vi "Do.vi"(8 "error in":errorcluster, 10 "Actor in":refnum<class "Actor.lvclass">, 11 "Update Device Configuration MSG":refnum<class "Update Device Configuration MSG.lvclass">) -> (0 "error out":errorcluster, 2 "Actor out":refnum<class "Actor.lvclass">)   [LabVIEW 2014, in "Controller.lvlib" / "Update Device Configuration MSG.lvclass"]
doc: "(<B>Filename</B>: Actor Framework.lvlib:Message.lvclass:Do.vi)\n\nDefines what a message does when it is received by an actor. Generally, a message instructs an actor to invoke one of its methods. By default, this method does nothing. A child class must override it to define behavior. Create a child class by using the Actor Framework Message Maker dialog box."
uses:
  Update Device Configuration MSG.lvclass
  <vilib>/ActorFramework/Actor/Actor.lvclass
  Controller.lvclass
  SuperActor/Ex Nested.lvclass/Ex Nested.ctl
  SuperActor/Read CVT Session.vi
  SuperActor/Read Log Session.vi
  <userlib>/_Session Fwk/Session - Root.lvclass
  reusable/Session APIs/Session Log/System Log.lvclass
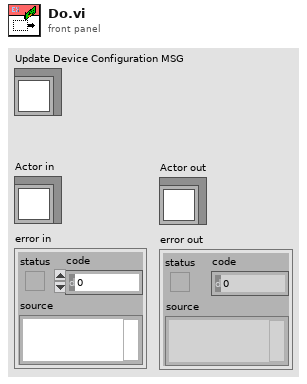
[diagram p1: front panel]
types:
  T1 = typedef "Session - Root.lvclass/Session Handle.ctl" = refnum<data-value>
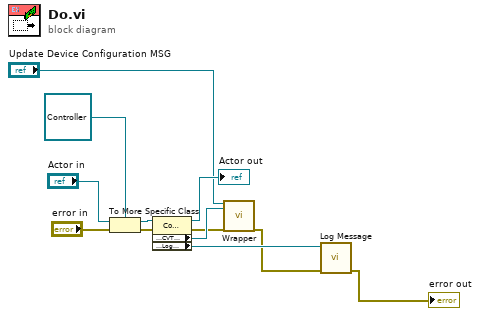
[diagram p0: block diagram]
diagram:
  n1 = To More Specific Class(target class=refnum<class "Controller.lvclass"> refnum ("Controller:Controller"), reference="Actor in", error in="error in") -> (specific class reference=w9:refnum<class "Controller.lvclass">, error out=w6:errorcluster)
  n2 = property class="Controller"(reference=w9, error in=w6) -> (reference out=→"Actor out":refnum<class "Controller.lvclass">, error out=w4:errorcluster, "Accessors:CVT Session"=w5:T1, "Accessors:Log Session"=w3:T1)
  n3 = call "Wrapper.vi"("Update Device Configuration in"="Update Device Configuration MSG", "CVT Session"=w5, "error in"=w4) -> ("error out"=w2:errorcluster)  [unwired: 16 in]
  n4 = call "Log Message.vi"("error in"=w2, "session in"=w3) -> ("error out"=→"error out":errorcluster)  [unwired: 8 in, 1 out]
